vi "DB update example.vi"(8 "error in (no error)":errorcluster) -> (0 "error out":errorcluster)   [LabVIEW 2012]
uses:
  Nick's small accelerator db/nick typedef.ctl
  <vilib>/addons/database/NI_Database_API.lvlib
panel:
  in  "Update data cluster":T1
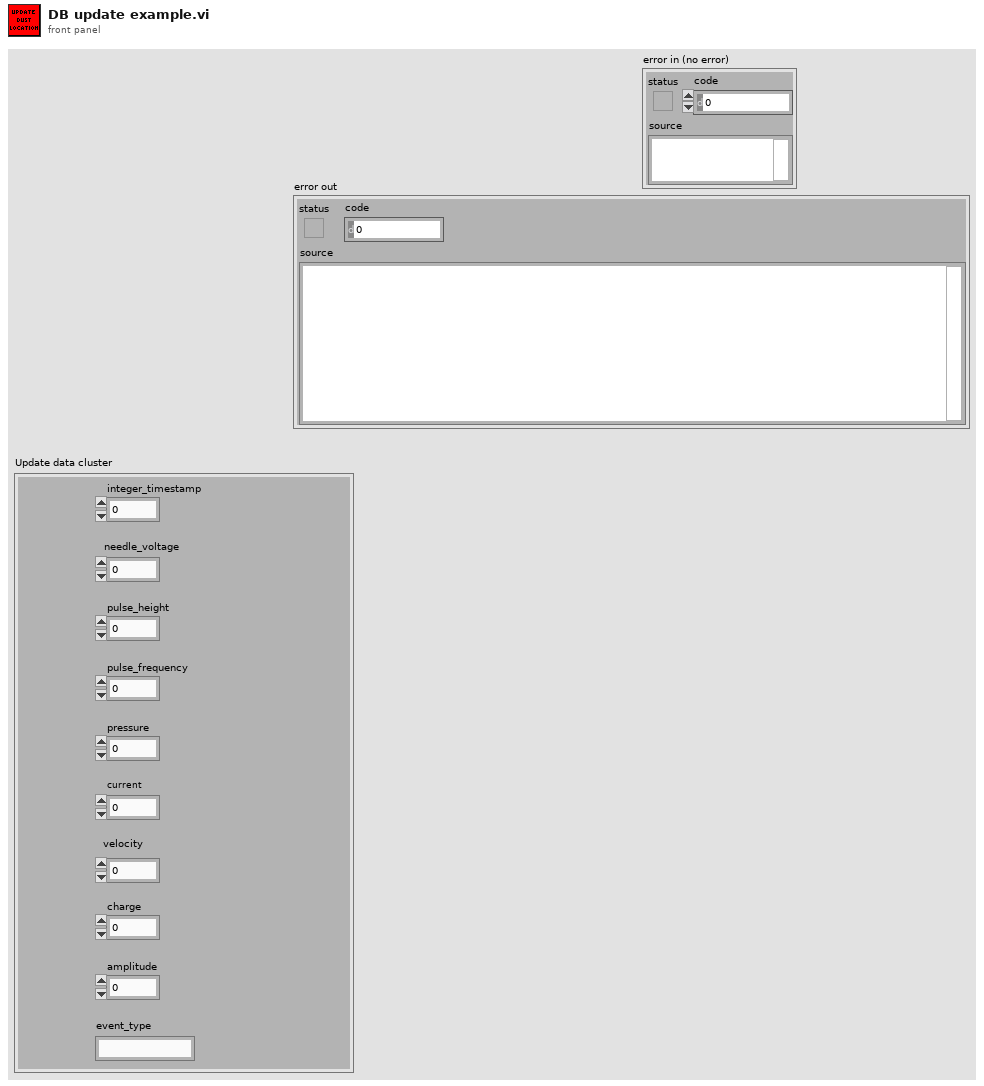
[diagram p1: front panel]
types:
  T1 = typedef "nick typedef.ctl" = cluster{"integer_timestamp":i64, "needle_voltage":dbl, "pulse_height":dbl, "pulse_frequency":dbl, "pressure":dbl, "current":dbl, "velocity":dbl, "charge":dbl, "amplitude":dbl, "event_type":string}
  T2 = typedef "NI_Database_API.lvlib/Conn ObjectReference.ctl" = refnum<k1>
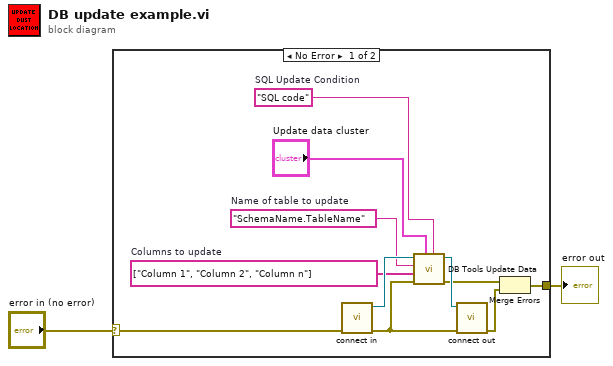
[diagram p0: block diagram]
diagram:
  n1 = case shown="No Error" "error in (no error)" {
    selector: "error in (no error)" -> [w12 w14]
    tunnel: [w9 w14] -> w1
    frame No Error {
      w3 = string[] ["Column 1", "Column 2", "Column n"]  # Columns to update
      w4 = "SchemaName.TableName"  # Name of table to update
      w5 = "SQL code"  # SQL Update Condition
      n2 = call "connect in.vi"("error in (no error)"=w12) -> ("error out"=w11:errorcluster, "Database Connection"=w13:T2)  [unwired: 6 in, 1 out]
      n3 = call <vilib>:"DB Tools Update Data.vi"("condition"=w5, "data"="Update data cluster", "error in (no error)"=w11, "columns"=w3, "table"=w4, "connection reference"=w13) -> ("error out"=w7:errorcluster, "connection reference out"=w8:T2)  [unwired: 4 in]
      n4 = call "connect out.vi"("error in (no error)"=w11, "connection reference"=w8) -> ("error out"=w10:errorcluster)  [unwired: 9 in]
      n5 = Merge Errors(w7, w10) -> (w9:errorcluster)
    }
    frame Error {
    }
  }
  "error out" <- w1
